vi "detOf3X3.vi"(1 "3x3 matrix":dbl[][](array[numeric])) -> (0 "Determinant":dbl)   [LabVIEW 2015]
doc: "3x3 array -- It's a 3x3 aray type.\nDeterminant -- The determinant of the 3x3 matrix."
panel:
  in  "stop":bool
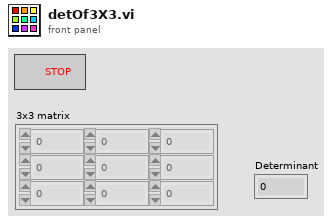
[diagram p1: front panel]
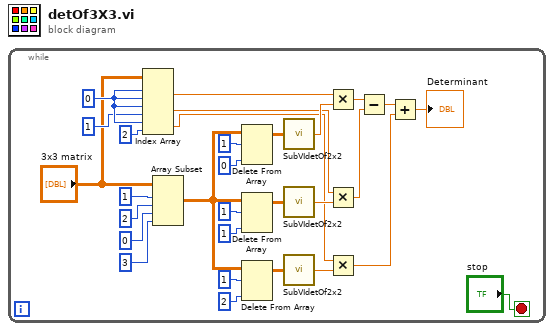
[diagram p0: block diagram]
diagram:
  n1 = while {
    stop <- "stop" stop-if-true
    w30 = 0 ("index (row)")
    n2 = Index Array(array="3x3 matrix", index (row) #1=w30, index (col) #1=w30, index (row) #2=w30, index (col) #2=1 ("disabled index (col)"), index (row) #3=w30, index (col) #3=2 ("disabled index (col)")) -> (element #1=w14:dbl, element #2=w12:dbl, element #3=w9:dbl)
    n3 = Array Subset(array="3x3 matrix", index (row)=1 ("index"), length (row)=2 ("length"), index (col)=0 ("index"), length (col)=3 ("length")) -> (w16:dbl[][])
    n4 = Delete From Array(array=w16, length=1, index (col)=0 ("disabled index (col)")) -> (array with subset deleted=w15:dbl[][])  [unwired: 1 in, 1 out]
    n5 = Delete From Array(array=w16, length=1, index (col)=1 ("disabled index (col)")) -> (array with subset deleted=w11:dbl[][])  [unwired: 1 in, 1 out]
    n6 = Delete From Array(array=w16, length=1, index (col)=2 ("disabled index (col)")) -> (array with subset deleted=w8:dbl[][])  [unwired: 1 in, 1 out]
    n7 = call "SubVIdetOf2x2.vi"("2x2Matrix"=w15) -> ("Determinant"=w13:dbl)
    n8 = call "SubVIdetOf2x2.vi"("2x2Matrix"=w11) -> ("Determinant"=w10:dbl)
    n9 = call "SubVIdetOf2x2.vi"("2x2Matrix"=w8) -> ("Determinant"=w7:dbl)
    n10 = Multiply(x=w14, y=w13) -> (x*y=w6:dbl)
    n11 = Multiply(x=w12, y=w10) -> (x*y=w5:dbl)
    n12 = Multiply(x=w9, y=w7) -> (x*y=w3:dbl)
    n13 = Subtract(x=w6, y=w5) -> (x-y=w4:dbl)
    n14 = Add(x=w4, y=w3) -> (x+y=→"Determinant":dbl)
  }
